vi "File Dialog.vi"(8 "error in (no error)":errorcluster, 10 "Overwrite?":bool, 11 "Path In":path) -> (0 "error out":errorcluster, 3 "Path Out":path)   [LabVIEW 2013]
doc: "File Dialog\n\nIf the path is not valid, this VI displays a File dialog box to choose the name of a new file.\n\n\n\nVersion 1.0\nDeveloped by Jean-Marc Simard\nCopyright © 2010, Exaprom Inc.\nAll rights reserved.\nLicense: BSD"
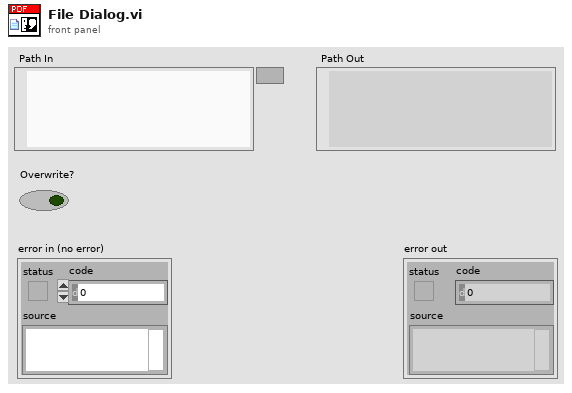
[diagram p1: front panel]
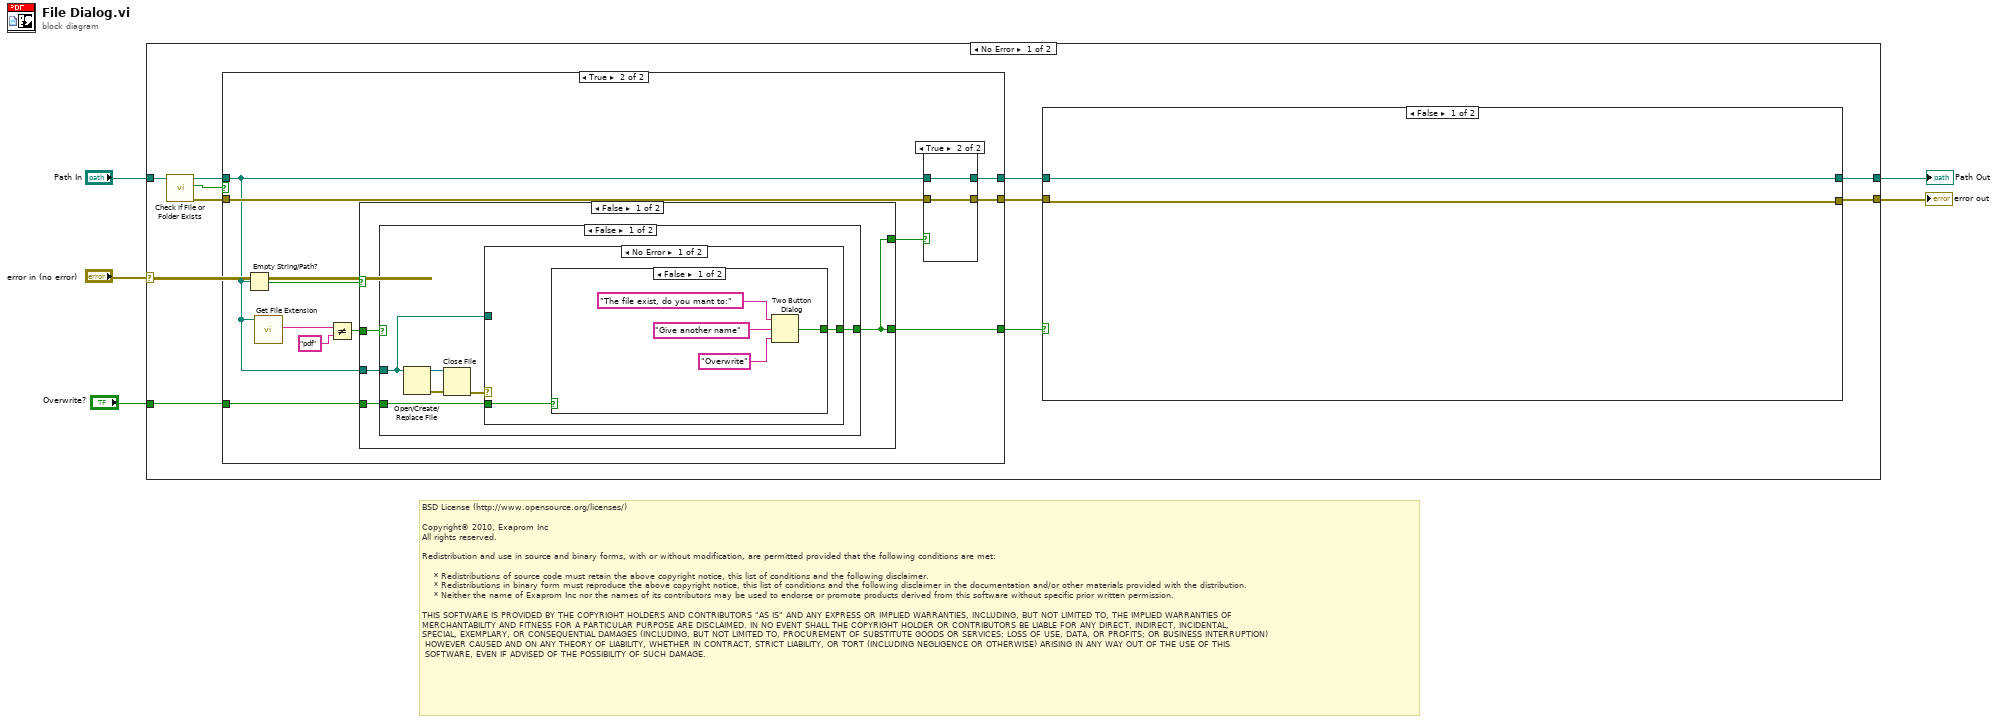
[diagram p0: block diagram]
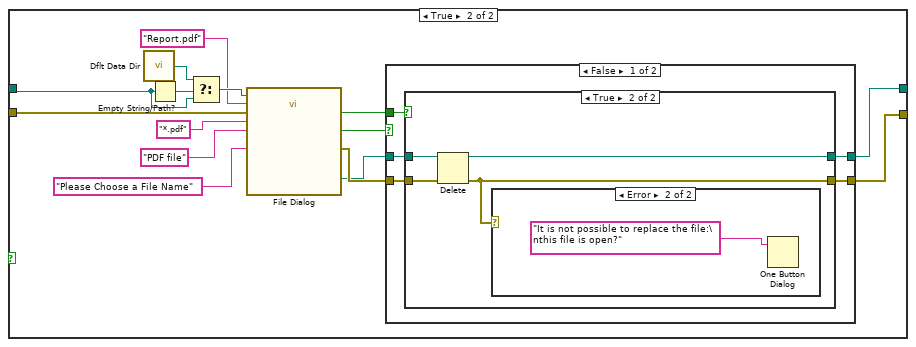
[diagram p2: hidden frame]
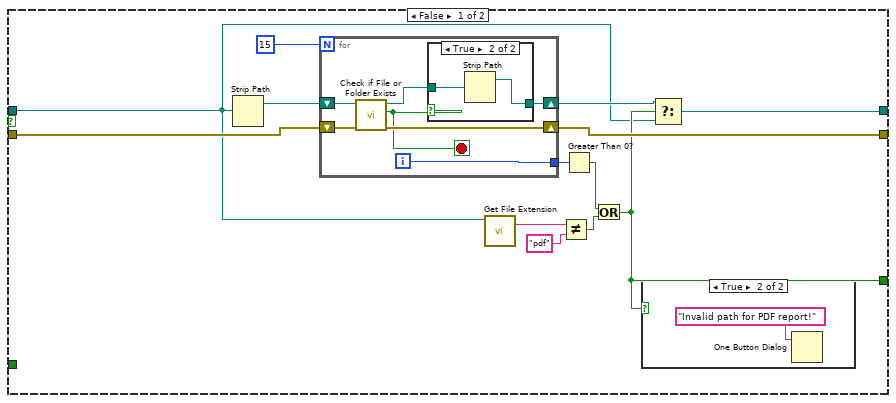
[diagram p6: hidden frame]
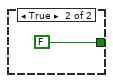
[diagram p9: hidden frame]
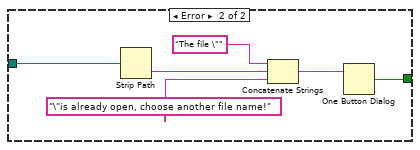
[diagram p10: hidden frame]
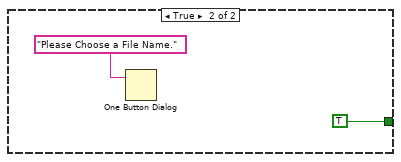
[diagram p11: hidden frame]
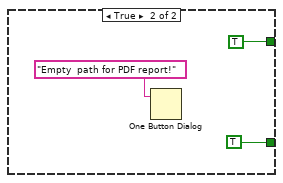
[diagram p12: hidden frame]
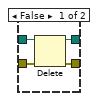
[diagram p13: hidden frame]
diagram:
  # "BSD License (http://www.opensource.org/licenses/)\n\nCopyright© 2010, Exaprom Inc\nAll rights reserved.\n\nRedistribution and use in source and binary forms, with or without modification, are permitted provided that the following conditions are met:\n\n    * Redistributions of source code must retain the above copyright notice, this list of conditions and the following disclaimer.\n    * Redistributions in binary form must reproduce the above copyright notice, this list of conditions and the following disclaimer in the documentation and/or other materials provided with the distribution.\n    * Neither the name of Exaprom Inc nor the names of its contributors may be used to endorse or promote products derived from this software without specific prior written permission.\n\nTHIS SOFTWARE IS PROVIDED BY THE COPYRIGHT HOLDERS AND CONTRIBUTORS \"AS IS\" AND ANY EXPRESS OR IMPLIED WARRANTIES, INCLUDING, BUT NOT LIMITED TO, THE IMPLIED WARRANTIES OF \nMERCHANTABILITY AND FITNESS FOR A PARTICULAR PURPOSE ARE DISCLAIMED. IN NO EVENT SHALL THE COPYRIGHT HOLDER OR CONTRIBUTORS BE LIABLE FOR ANY DIRECT, INDIRECT, INCIDENTAL,\nSPECIAL, EXEMPLARY, OR CONSEQUENTIAL DAMAGES (INCLUDING, BUT NOT LIMITED TO, PROCUREMENT OF SUBSTITUTE GOODS OR SERVICES; LOSS OF USE, DATA, OR PROFITS; OR BUSINESS INTERRUPTION)\n HOWEVER CAUSED AND ON ANY THEORY OF LIABILITY, WHETHER IN CONTRACT, STRICT LIABILITY, OR TORT (INCLUDING NEGLIGENCE OR OTHERWISE) ARISING IN ANY WAY OUT OF THE USE OF THIS\n SOFTWARE, EVEN IF ADVISED OF THE POSSIBILITY OF SUCH DAMAGE."
  n1 = case shown="No Error" "error in (no error)" {
    selector: "error in (no error)" -> [_ w117]
    tunnel: [w9 w117] -> w5
    tunnel: "Path In" -> [w8 w116]
    tunnel: [w10 w116] -> w2
    tunnel: "Overwrite?" -> [w6 _]
    frame No Error {
      n2 = call <vilib>:"Check if File or Folder Exists.vi"("path"=w8) -> ("error out"=w14:errorcluster, "file or folder exists?"=w15:bool, "dup path"=w7:path)  [unwired: 1 in, 7 out]
      n3 = case shown="True" w15 {
        tunnel: w7 -> [w48 w73]
        tunnel: [w50 w81] -> w12
        tunnel: w14 -> [w54 w79]
        tunnel: [w55 w80] -> w11
        tunnel: [w51 w78] -> w13
        tunnel: w6 -> [_ w71]
        frame False {
          n4 = Strip Path(path=w48) -> (stripped path=w59:path)  [unwired: 1 out]
          n5 = for {
            N: 15 -> [_]
            shift-right: [w65] -> w49
            shift-left: w59 -> [w67]
            tunnel: [w64] -> w56
            shift-right: [w63] -> w55
            shift-left: w54 -> [w62]
            i -> [w64]
            stop <- w61 stop-if-true
            n6 = call <vilib>:"Check if File or Folder Exists.vi"("error in (no error)"=w62, "path"=w67) -> ("error out"=w63:errorcluster, "file or folder exists?"=w61:bool, "dup path"=w66:path)  [unwired: 7 out]
            n7 = case shown="True" w61 {
              tunnel: w66 -> [w68 w70]
              tunnel: [w68 w69] -> w65
              frame False {
              }
              frame True {
                n8 = Strip Path(path=w70) -> (stripped path=w69:path)  [unwired: 1 out]
              }
            }
          }
          n9 = call <vilib>:"Get File Extension.vi"("file"=w48) -> ("lowercase file extension"=w47:string)  [unwired: 1 in, 9 out]
          n10 = Not Equal?(x=w47, y="pdf") -> (x != y?=w53:bool)
          n11 = Greater Than 0?(x=w56) -> (x > 0?=w52:bool)
          n12 = Or(x=w52, y=w53) -> (x .or. y?=w51:bool)
          n13 = case shown="True" w51 {
            frame False {
            }
            frame True {
              n14 = One Button Dialog(message="Invalid path for PDF report!") -> ()  [unwired: 2 out]
            }
          }
          n15 = Select(t=w49, s=w51, f=w48) -> (s? t:f=w50:path)
        }
        frame True {
          n16 = Empty String/Path?(string/path=w73) -> (empty?=w77:bool)
          n17 = call <vilib>:"Get File Extension.vi"("file"=w73) -> ("lowercase file extension"=w72:string)  [unwired: 1 in, 9 out]
          n18 = Not Equal?(x=w72, y="pdf") -> (x != y?=w74:bool)
          n19 = case shown="False" w77 {
            tunnel: [w85 TRUE ("T button?")] -> w78
            tunnel: [w85 TRUE] -> w76
            tunnel: w74 -> [w84 _]
            tunnel: w73 -> [w83 _]
            tunnel: w71 -> [w82 _]
            frame False {
              n20 = case shown="False" w84 {
                tunnel: [w91 TRUE] -> w85
                tunnel: w83 -> [w87 _]
                tunnel: w82 -> [w86 _]
                frame False {
                  n21 = Open/Create/Replace File(file path (use dialog)=w87) -> (refnum out=w89:refnum<file>, error out=w90:errorcluster)  [unwired: 1 in, 5 out]
                  n22 = Close File(refnum=w89, error in=w90) -> (error out=w88:errorcluster)  [unwired: 1 out]
                  n23 = case shown="No Error" w88 {
                    tunnel: [w93 w104] -> w91
                    tunnel: w87 -> [_ w99]
                    tunnel: w86 -> [w92 _]
                    frame No Error {
                      n24 = case shown="False" w92 {
                        tunnel: [w94 FALSE] -> w93
                        frame False {
                          n25 = Two Button Dialog(message="The file exist, do you mant to:", 1:"Overwrite" ("T button name (\"OK\")"), 2:"Give another name" ("F button name (\"Cancel\")")) -> (T button?=w94:bool)
                        }
                        frame True {
                        }
                      }
                    }
                    frame Error {
                      n26 = Strip Path(path=w99) -> (name=w102:string)  [unwired: 1 out]
                      n27 = Concatenate Strings("The file \"", w102, "\"is already open, choose another file name!") -> (w100:string)
                      n28 = One Button Dialog(message=w100) -> (true=w104:bool)  [unwired: 1 out]
                    }
                  }
                }
                frame True {
                  n29 = One Button Dialog(message="Please Choose a File Name." ("prompt")) -> ()  [unwired: 2 out]
                }
              }
            }
            frame True {
              n30 = One Button Dialog(message="Empty  path for PDF report!") -> ()  [unwired: 2 out]
            }
          }
          n31 = case shown="True" w76 {
            tunnel: [w113 w115] -> w81
            tunnel: [w112 w114] -> w80
            tunnel: w79 -> [w111 w114]
            tunnel: w73 -> [w110 w115]
            frame False {
              n32 = Delete(path (use dialog)=w110, error in=w111) -> (deleted path=w113:path, error out=w112:errorcluster)  [unwired: 4 out]
            }
            frame True {
            }
          }
        }
      }
      n33 = case shown="False" w13 {
        tunnel: w12 -> [w17 w28]
        tunnel: [w17 w20] -> w10
        tunnel: w11 -> [w16 w31]
        tunnel: [w16 w21] -> w9
        frame False {
        }
        frame True {
          n34 = call <vilib>:"Dflt Data Dir.vi"() -> ("App:Default Data Directory"=w19:path)
          n35 = Empty String/Path?(string/path=w28) -> (empty?=w29:bool)
          n36 = Select(t=w19, s=w29, f=w28) -> (s? t:f=w27:path)
          n37 = call "File Dialog"("start path"=w27, "prompt"="Please Choose a File Name", "default name"="Report.pdf", "error in"=w31, "pattern (all files)"="*.pdf", "pattern label"="PDF file") -> ("selected path"=w22:path, "exists"=w24:bool, "cancelled"=w25:bool, "error out"=w23:errorcluster)  [unwired: 1 in, 5 out]
          n38 = case shown="False" w25 {
            tunnel: w24 -> [w37 _]
            tunnel: w23 -> [w36 w46]
            tunnel: w22 -> [w35 w45]
            tunnel: [w34 w46] -> w21
            tunnel: [w33 w45] -> w20
            frame False {
              n39 = case shown="True" w37 {
                tunnel: w36 -> [w38 w43]
                tunnel: w35 -> [w39 w42]
                tunnel: [w38 w40] -> w34
                tunnel: [w39 w41] -> w33
                frame False {
                }
                frame True {
                  n40 = Delete(path (use dialog)=w42, error in=w43) -> (deleted path=w41:path, error out=w40:errorcluster)  [unwired: 4 out]
                  n41 = case shown="Error" w40 {
                    frame No Error {
                    }
                    frame Error {
                      n42 = One Button Dialog(message="It is not possible to replace the file:\nthis file is open?" ("prompt")) -> ()  [unwired: 2 out]
                    }
                  }
                }
              }
            }
            frame True {
            }
          }
        }
      }
    }
    frame Error {
    }
  }
  "error out" <- w5
  "Path Out" <- w2
